vi "Write ChannelData.vi"(8 "error in (no error)":errorcluster, 10 "ChannelData":dbl[][](array[numeric]), 11 "EMG in":refnum<class "EMG.lvclass">) -> (0 "error out":errorcluster, 3 "EMG out":refnum<class "EMG.lvclass">)   [LabVIEW 2014, in "EMG.lvclass"]
uses:
  EMG.lvclass
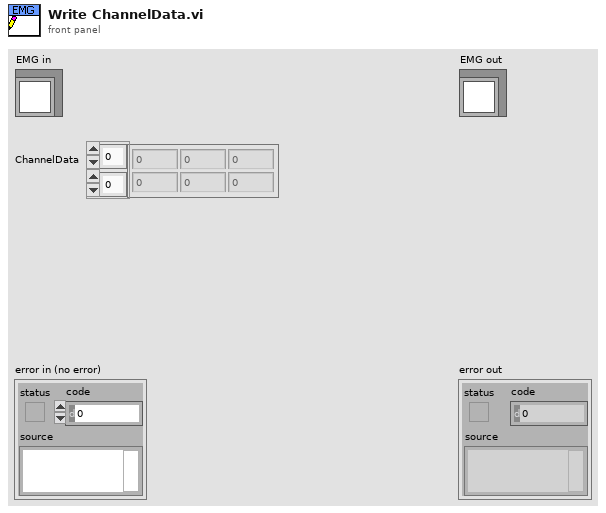
[diagram p1: front panel]
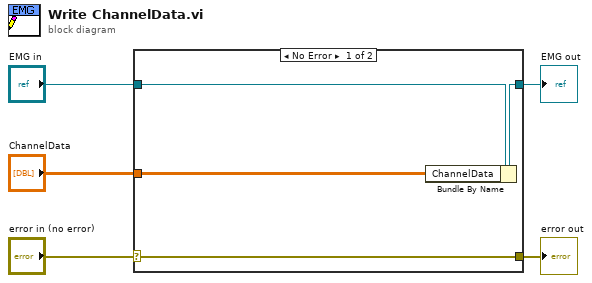
[diagram p0: block diagram]
diagram:
  n1 = case shown="No Error" "error in (no error)" {
    selector: "error in (no error)" -> [w9 w10]
    tunnel: [w9 w10] -> w4
    tunnel: [w7 w11] -> w2
    tunnel: "EMG in" -> [w8 w11]
    tunnel: "ChannelData" -> [w6 _]
    frame No Error {
      n2 = Bundle By Name(cluster=w8, "ChannelData"=w6) -> (w7:refnum<class "EMG.lvclass">)
    }
    frame Error {
    }
  }
  "error out" <- w4
  "EMG out" <- w2
